vi "PM100D_Read.vi"(3 "error in (no error)":errorcluster, 4 "Command":string, 6 "VISA in":refnum<visa-resource-name>="COM1") -> (0 "error out":errorcluster, 1 "ReadValue":string, 2 "VISA out":refnum<visa-resource-name>)   [LabVIEW 2014]
doc: "Reads data from the connected instrument. All query commands according the SCPI command table are terminated by a question mark (?)"
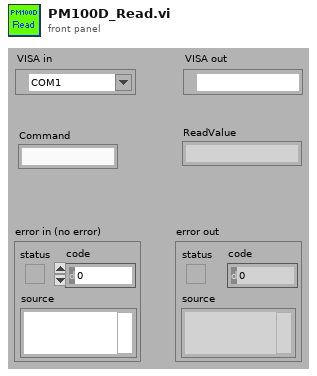
[diagram p1: front panel]
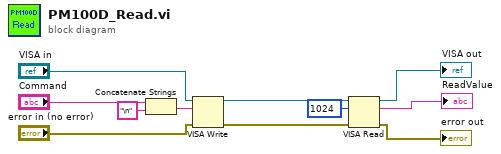
[diagram p0: block diagram]
diagram:
  n1 = Concatenate Strings("Command", "\n" ("String")) -> (w8:string)
  n2 = VISA Write(VISA resource name="VISA in", write buffer=w8, error in (no error)="error in (no error)") -> (VISA resource name out=w6:refnum<visa-resource-name>, error out=w3:errorcluster)  [unwired: 1 out]
  n3 = VISA Read(VISA resource name=w6, byte count=u32 1024, error in (no error)=w3) -> (VISA resource name out=→"VISA out":refnum<visa-resource-name>, read buffer=→"ReadValue":string, error out=→"error out":errorcluster)  [unwired: 1 out]
